vi "CoboldState.vi"(0 "Strings in":string[](array[string])=["C:\\CuspControl\\GPIB and Network\\Cusp\\CoboldState.txt", "6723"], 1 "Dubs in":dbl[](array[numeric])=[0.0, 0.0]) -> ()   [LabVIEW 2018]
panel:
  in  "Run Duration (s)":dbl
  in  "subvi":bool=TRUE
  in  "Cobold State":dbl
  in  "Slave File":path=path "C:/CuspControl/GPIB and Network/Cusp/CoboldState.txt"
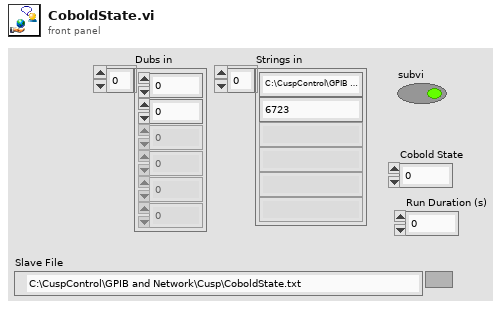
[diagram p1: front panel]
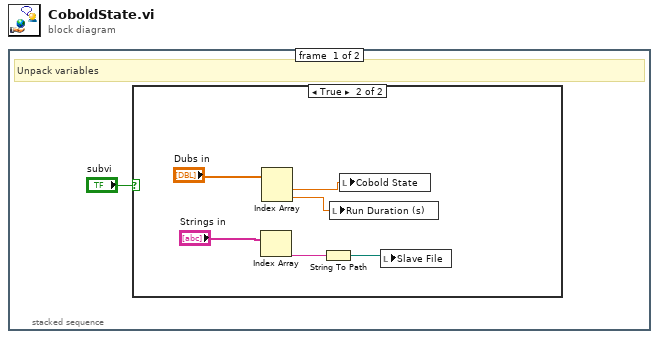
[diagram p0: block diagram]
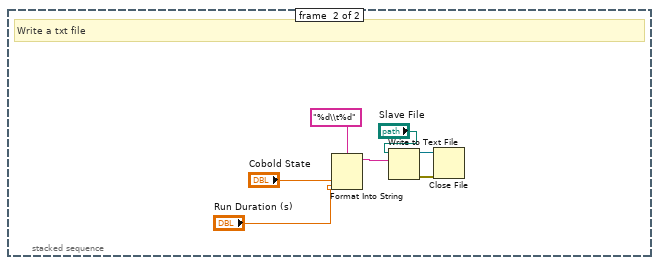
[diagram p3: hidden frame]
diagram:
  n1 = stacked-sequence {
    frame #0 {
      # "Unpack variables"
      n2 = case shown="True" "subvi" {
        frame False {
        }
        frame True {
          n3 = Index Array(array="Strings in") -> (element=w4:string)  [unwired: 1 in]
          n4 = Index Array(array="Dubs in") -> (element #1=w5:dbl, element #2=w2:dbl)  [unwired: 2 in]
          n5 = String To Path(string=w4) -> (path=w3:path)
          n6 = local write "Run Duration (s)"(w2) -> ()
          n7 = local write "Cobold State"(w5) -> ()
          n8 = local write "Slave File"(w3) -> ()
        }
      }
    }
    frame #1 {
      # "Write a txt file"
      n9 = Format Into String(format string="%d\\t%d", "Cobold State", "Run Duration (s)") -> (resulting string=w13:string)  [unwired: 2 in, 1 out]
      n10 = Write to Text File(file (use dialog)="Slave File", text=w13) -> (refnum out=w9:refnum<file>, error out=w10:errorcluster)  [unwired: 2 in, 1 out]
      n11 = Close File(refnum=w9, error in=w10) -> ()  [unwired: 2 out]
    }
  }
